vi "LaunchNested.vi"(8 "error in (no error)":errorcluster, 11 "Caller in":refnum<class "Caller.lvclass">) -> (0 "error out":errorcluster, 3 "Caller out":refnum<class "Caller.lvclass">)   [LabVIEW 2020, in "Caller.lvlib" / "Caller.lvclass"]
uses:
  Caller.lvclass
  C:/Program Files/National Instruments/LabVIEW 2020/vi.lib/ActorFramework/Actor/Actor.lvclass
  Nested/Nested.lvclass
  Caller.lvclass/Caller.ctl
  <vilib>/ActorFramework/Actor/Actor.lvclass
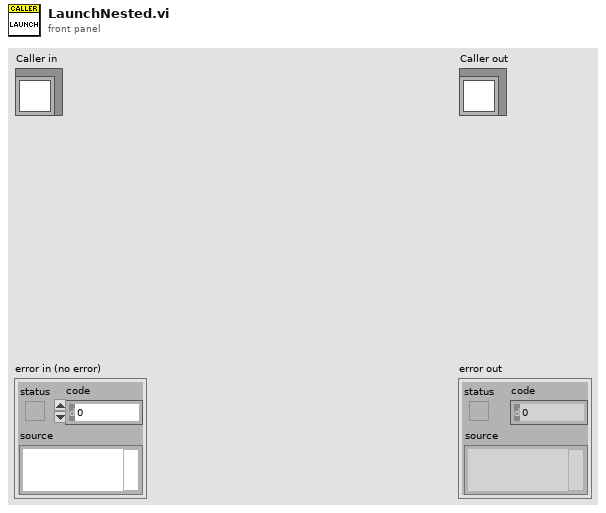
[diagram p1: front panel]
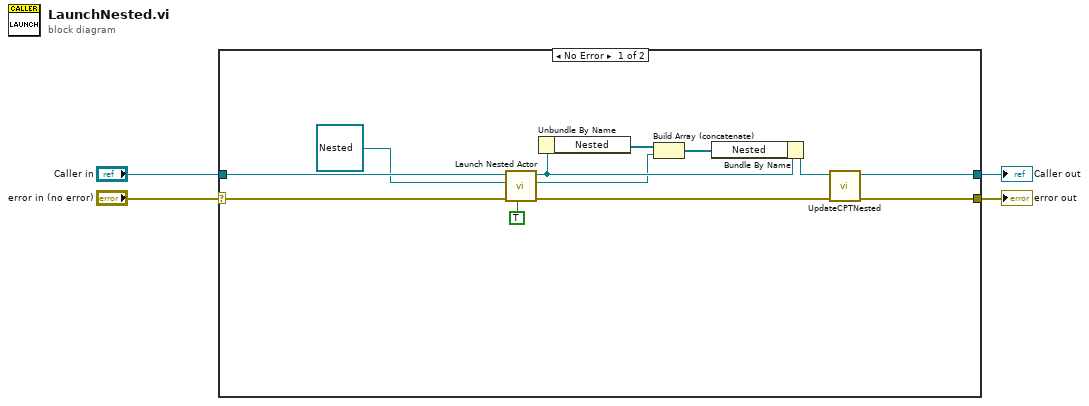
[diagram p0: block diagram]
diagram:
  n1 = case shown="No Error" "error in (no error)" {
    selector: "error in (no error)" -> [w15 w18]
    tunnel: [w11 w18] -> w3
    tunnel: [w10 w17] -> w1
    tunnel: "Caller in" -> [w16 w17]
    frame No Error {
      n2 = call <vilib>:"Launch Nested Actor.vi"("Open Actor Core front panel? (F)"=TRUE, "error in (no error)"=w15, "Nested Actor"=refnum<class "Nested.lvclass"> refnum ("Nested.lvlib:Nested.lvclass"), "Caller Actor in"=w16) -> ("error out"=w12:errorcluster, "Nested Actor's Enqueuer"=w5:refnum<class "Message Enqueuer.lvclass">, "Caller Actor out"=w9:refnum<class "Caller.lvclass">)  [unwired: 5 in]
      n3 = Unbundle By Name(w9) -> ("Nested"=w7:refnum<class "Message Enqueuer.lvclass">[])
      n4 = Build Array (concatenate)(w7, w5) -> (w6:refnum<class "Message Enqueuer.lvclass">[])
      n5 = Bundle By Name(cluster=w9, "Nested"=w6) -> (w8:refnum<class "Caller.lvclass">)
      n6 = call "UpdateCPTNested.vi"("error in (no error)"=w12, "Caller in"=w8) -> ("error out"=w11:errorcluster, "Caller out"=w10:refnum<class "Caller.lvclass">)  [unwired: 8 in]
    }
    frame Error {
    }
  }
  "error out" <- w3
  "Caller out" <- w1
